vi "SplitterNoisePowerCheckSingle.vi"(3 "error in (no error)":errorcluster) -> (0 "error out":errorcluster, 1 "String_PNG_Amp_Split":string, 2 "dBAvg Noise Power to splitter (dBm)":dbl format="%.3f", 5 "dBSSD Noise Power to splitter (dB)":dbl format="%.3f")   [LabVIEW 2009]
doc: "Test out attenuation switching with inside noise source"
panel:
  out "dBPeakToAver (dB)":dbl format="%.5f"
  in  "Select_Interval_between_readings mS":i32=50 min=1 max=1000 step=1
  out "LinAvg Noise Power to splitter (dBm)":dbl format="%.3f"
  in  "Select NreadingsFromPwrMeterToAverage":i32=30 min=1 max=1000 step=1
  # "Insure that the correct power meter averaging mode is set up prior to this call."
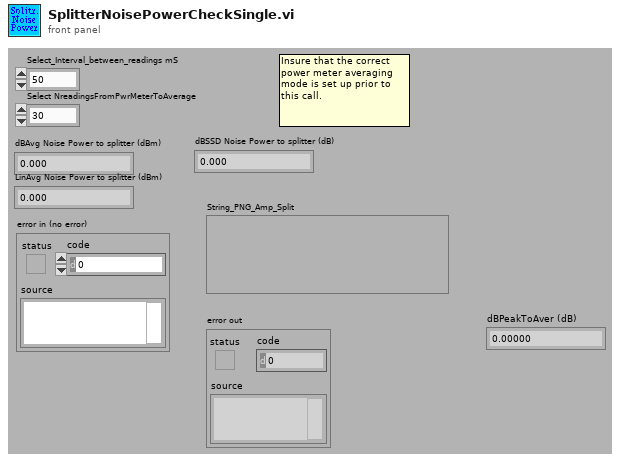
[diagram p1: front panel]
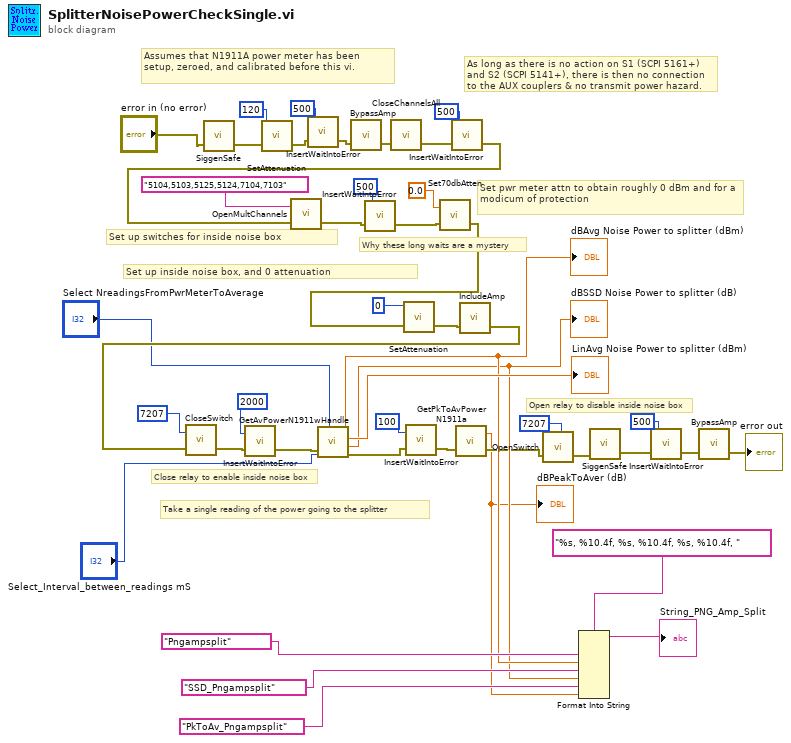
[diagram p0: block diagram]
diagram:
  # "As long as there is no action on S1 (SCPI 5161+) and S2 (SCPI 5141+), there is then no connection to the AUX couplers & no transmit power hazard."
  # "Assumes that N1911A power meter has been setup, zeroed, and calibrated before this vi."
  # "Why these long waits are a mystery"
  # "Open relay to disable inside noise box"
  # "Close relay to enable inside noise box"
  # "Set pwr meter attn to obtain roughly 0 dBm and for a modicum of protection"
  # "Set up switches for inside noise box"
  # "Take a single reading of the power going to the splitter"
  # "Set up inside noise box, and 0 attenuation"
  n1 = call "SiggenSafe.vi"("error in (no error)"="error in (no error)") -> ("error out"=w22:errorcluster)  [unwired: 2 in]
  n2 = call "SetAttenuation.vi"("error in (no error)"=w22, "Attenuation (dB)"=120) -> ("error out"=w19:errorcluster)  [unwired: 1 in]
  n3 = call "InsertWaitIntoError.vi"("error in (no error)"=w19, "Wait (msecs)"=500) -> ("error out"=w18:errorcluster)  [unwired: 1 in]
  n4 = call "BypassAmp.vi"("error in (no error)"=w18) -> ("error out"=w39:errorcluster)  [unwired: 2 in]
  n5 = call "CloseChannelsAll.vi"("error in (no error)"=w39) -> ("error out"=w41:errorcluster)  [unwired: 2 in]
  n6 = call "InsertWaitIntoError.vi"("error in (no error)"=w41, "Wait (msecs)"=500) -> ("error out"=w36:errorcluster)  [unwired: 1 in]
  n7 = call "OpenMultChannels.vi"("error in (no error)"=w36, "Channels to be opened"="5104,5103,5125,5124,7104,7103") -> ("error out"=w25:errorcluster)  [unwired: 1 in]
  n8 = call "InsertWaitIntoError.vi"("error in (no error)"=w25, "Wait (msecs)"=500) -> ("error out"=w24:errorcluster)  [unwired: 1 in]
  n9 = call "Set70dbAtten.vi"("error in (no error)"=w24, "Attenuation (dB)"=0.0) -> ("error out"=w32:errorcluster)  [unwired: 1 in]
  n10 = call "SetAttenuation.vi"("error in (no error)"=w32, "Attenuation (dB)"=0) -> ("error out"=w37:errorcluster)  [unwired: 1 in]
  n11 = call "IncludeAmp.vi"("error in (no error)"=w37) -> ("error out"=w30:errorcluster)  [unwired: 2 in]
  n12 = call "CloseSwitch.vi"("error in (no error)"=w30, "Switch ID"=7207) -> ("error out"=w29:errorcluster)  [unwired: 1 in]
  n13 = call "InsertWaitIntoError.vi"("error in (no error)"=w29, "Wait (msecs)"=2000) -> ("error out"=w33:errorcluster)  [unwired: 1 in]
  n14 = call "GetAvPowerN1911wHandle.vi"("error in (no error)"=w33, "NreadingsFromPwrMeter"="Select NreadingsFromPwrMeterToAverage", "IntervalBetweenReadings (mS)"="Select_Interval_between_readings mS") -> ("Error out"=w4:errorcluster, "VI dBSSD Power (dB)"=w9:dbl, "Computed LinMean Power (dBm)"=→"LinAvg Noise Power to splitter (dBm)":dbl, "VI dBMean Power (dBm)"=w10:dbl)  [unwired: 2 in, 3 out]
  "dBAvg Noise Power to splitter (dBm)" <- w10
  "dBSSD Noise Power to splitter (dB)" <- w9
  n15 = call "InsertWaitIntoError.vi"("error in (no error)"=w4, "Wait (msecs)"=100) -> ("error out"=w5:errorcluster)  [unwired: 1 in]
  n16 = call "GetPkToAvPowerN1911a.vi"("error in (no error)"=w5) -> ("Error out"=w3:errorcluster, "Power returned (dBm)"=w1:dbl)  [unwired: 1 in]
  "dBPeakToAver (dB)" <- w1
  n17 = call "OpenSwitch.vi"("error in (no error)"=w3, "Switch ID"=7207) -> ("error out"=w27:errorcluster)  [unwired: 1 in]
  n18 = Format Into String(format string="%s, %10.4f, %s, %10.4f, %s, %10.4f, ", "Pngampsplit", w10, "SSD_Pngampsplit", w9, "PkToAv_Pngampsplit", w1) -> (resulting string=→"String_PNG_Amp_Split":string)  [unwired: 2 in, 1 out]
  n19 = call "SiggenSafe.vi"("error in (no error)"=w27) -> ("error out"=w17:errorcluster)  [unwired: 2 in]
  n20 = call "InsertWaitIntoError.vi"("error in (no error)"=w17, "Wait (msecs)"=500) -> ("error out"=w16:errorcluster)  [unwired: 1 in]
  n21 = call "BypassAmp.vi"("error in (no error)"=w16) -> ("error out"=→"error out":errorcluster)  [unwired: 2 in]
